vi "LogToXMLFile.vi"(8 "Error In":errorcluster, 11 "LogClassData In":refnum<class "LogClassData.lvclass">) -> (0 "Error Out":errorcluster, 3 "LogClassData Out":refnum<class "LogClassData.lvclass">)   [LabVIEW 2021, in "LogClassData.lvclass"]
doc: "Save specific class data to file as XML."
uses:
  LogClassData.lvclass
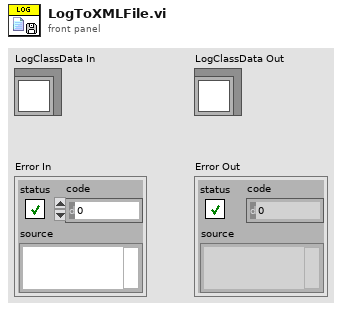
[diagram p1: front panel]
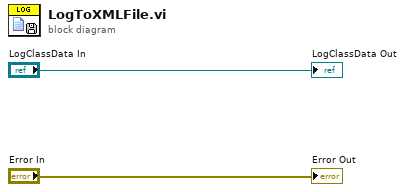
[diagram p0: block diagram]
diagram:
  "Error Out" <- "Error In"
  "LogClassData Out" <- "LogClassData In"
